vi "compare aggregates is and for equals.vi"() -> ()   [LabVIEW 2010]
panel:
  out "x = y?":bool
  in  "Array 2":u32[](array[numeric])
  in  "Array":u32[](array[numeric])
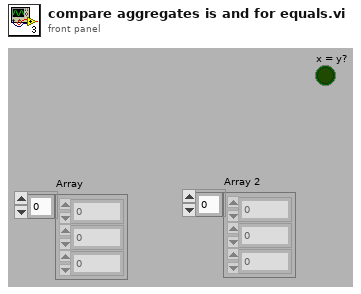
[diagram p1: front panel]
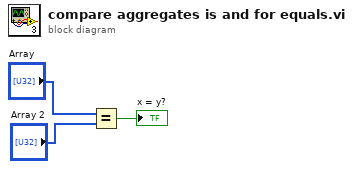
[diagram p0: block diagram]
diagram:
  n1 = Equal?(x="Array", y="Array 2") -> (x = y?=→"x = y?":bool)
